vi "Standard Event Register Query.vi"(0 "VISA resource name":refnum<visa-resource-name>, 11 "error in (no error)":errorcluster) -> (4 "VISA resource name out":refnum<visa-resource-name>, 6 "Event Status Register":T1, 15 "error out":errorcluster)   [LabVIEW 2018, in "XP Power PLS600.lvlib"]
doc: "Queries the Event Status Register and returns the byte data available in it.\nEach bit represent the occurrence of an event.\n\nEx : BIT 0 is set High when \"Operation Complete\"\n\nBIT 0: Operation Complete\nBIT 1: Request Control\nBIT 2: Query Error\nBIT 3: Device Error\nBIT 4: Execution Error\nBIT 5: Command Error\nBIT 6: User Request\nBIT 7: Power On"
uses:
  XP Power PLS600.lvlib
panel:
  # "BIT 0: Operation Complete\nBIT 1: Request Control\nBIT 2: Query Error\nBIT 3: Device Dependant Error\nBIT 4: Execution Error\nBIT 5: Command Error\nBIT 6: User Request\nBIT 7: Power On"
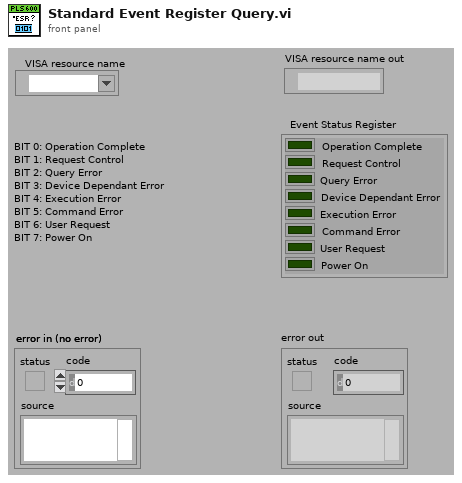
[diagram p1: front panel]
types:
  T1 = cluster{"Operation Complete":bool, "Request Control":bool, "Query Error":bool, "Device Dependant Error":bool, "Execution Error":bool, "Command Error":bool, "User Request":bool, "Power On":bool}
  T2 = cluster{"Boolean array[0]":bool, "Boolean array[1]":bool, "Boolean array[2]":bool, "Boolean array[3]":bool, "Boolean array[4]":bool, "Boolean array[5]":bool, "Boolean array[6]":bool, "Boolean array[7]":bool}
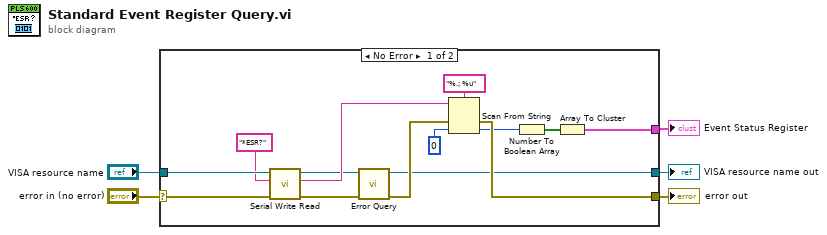
[diagram p0: block diagram]
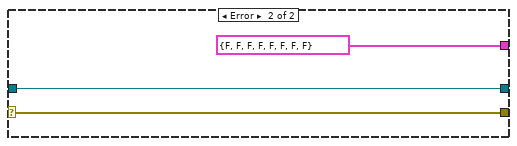
[diagram p2: hidden frame]
diagram:
  n1 = case shown="No Error" "error in (no error)" {
    selector: "error in (no error)" -> [w17 w22]
    tunnel: [w19 T2 {"Boolean array[0]"=FALSE, "Boolean array[1]"=FALSE, "Boolean array[2]"=FALSE, "Boolean array[3]"=FALSE, "Boolean array[4]"=FALSE, "Boolean array[5]"=FALSE, "Boolean array[6]"=FALSE, "Boolean array[7]"=FALSE} ("Boolean array")] -> w1
    tunnel: [w18 w22] -> w2
    tunnel: "VISA resource name" -> [w16 w21]
    tunnel: [w6 w21] -> w4
    frame No Error {
      n2 = call "Serial Write Read.vi"("error in (no error)"=w17, "Write Buffer"="*ESR?" ("Command to Send (empty)"), "VISA resource name"=w16) -> ("error out"=w8:errorcluster, "Read Buffer"=w10:string, "VISA resource name out"=w9:refnum<visa-resource-name>)  [unwired: 6 in]
      n3 = call "Error Query.vi"("error in (no error)"=w8, "VISA resource name"=w9) -> ("error out"=w7:errorcluster, "VISA resource name out"=w6:refnum<visa-resource-name>)  [unwired: 6 in, 2 out]
      n4 = Scan From String(format string="%.; %u" ("Format String"), input string=w10, error in=w7, default 1=u8 0 ("default value 1")) -> (error out=w18:errorcluster, output 1=w12:u8)  [unwired: 1 in, 2 out]
      n5 = Number To Boolean Array(number=w12) -> (Boolean array=w14:bool[])
      n6 = Array To Cluster(array=w14) -> (cluster=w19:T2)
    }
    frame Error {
    }
  }
  "Event Status Register" <- w1
  "VISA resource name out" <- w4
  "error out" <- w2
